vi "DRIVE_HDG_TARGET.vi"(10 "argv":string[](array[string]), 11 "args":u8) -> ()   [LabVIEW 2011]
uses:
  <vilib>/Rock Robotics/WPI/DriverStation/WPI_DriverStationStatusErrorCache.ctl
  Auto_Conf.vi
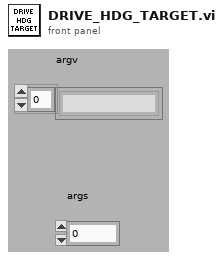
[diagram p1: front panel]
types:
  T1 = typedef "WPI_GyroDevRef.ctl" = cluster{"DevStatus":errorcluster, "Analog Module":T2, "Analog Channel":T3, "Offset":dbl, "Gain (VoltsPerDegree/Second)":dbl}
  T2 = typedef "FPGA_TypedefAnalogModule.ctl" = enum16{"Analog Module 1", "Analog Module 2"}
  T3 = typedef "FPGA_AIChannel.ctl" = enum8{"AI 1", "AI 2", "AI 3", "AI 4", "AI 5", "AI 6", "AI 7", "AI 8", "Invalid"}
  T4 = typedef "WPI_DriverStationStatusErrorCache.ctl" = enum16{"Get", "Set"}
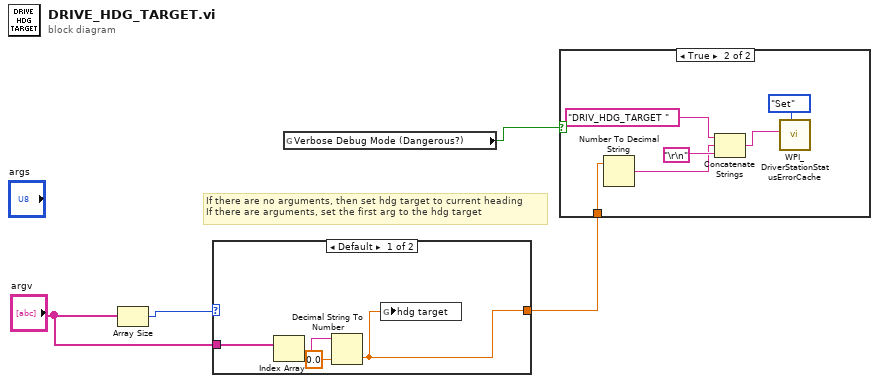
[diagram p0: block diagram]
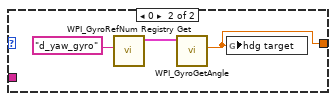
[diagram p3: hidden frame]
diagram:
  # "If there are no arguments, then set hdg target to current heading\nIf there are arguments, set the first arg to the hdg target"
  n1 = Array Size(array="argv") -> (size(s)=w1:i32)
  n2 = case shown="Default" w1 {
    tunnel: "argv" -> [w8 _]
    tunnel: [w5 w9] -> w3
    frame Default {
      n3 = Index Array(array=w8) -> (element=w7:string)  [unwired: 1 in]
      n4 = Decimal String To Number(string=w7, default (0L)=0.0 ("default (0 I32)")) -> (number=w5:dbl)  [unwired: 1 in, 1 out]
      n5 = global write "Auto_Conf.vi" "hdg target"(w5) -> ()
    }
    frame 0 {
      n6 = call <vilib>:"WPI_GyroRefNum Registry Get.vi"("refnum name"="d_yaw_gyro") -> ("GyroDevRef"=w10:T1)  [unwired: 1 in, 9 out]
      n7 = call <vilib>:"WPI_GyroGetAngle.vi"("GyroDevRef"=w10) -> ("Angle"=w9:dbl)  [unwired: 7 in, 3 out]
      n8 = global write "Auto_Conf.vi" "hdg target"(w9) -> ()
    }
  }
  n9 = global read "Auto_Conf.vi" "Verbose Debug Mode (Dangerous?)"() -> (w4:bool)
  n10 = case shown="True" w4 {
    tunnel: w3 -> [_ w12]
    frame False {
    }
    frame True {
      n11 = Number To Decimal String(number=w12) -> (decimal integer string=w13:string)  [unwired: 1 in]
      n12 = Concatenate Strings("DRIV_HDG_TARGET " ("string"), w13, "\r\n") -> (w15:string)
      n13 = call <vilib>:"WPI_DriverStationStatusErrorCache.vi"("StatusErrorCacheOp"=WPI_DriverStationStatusErrorCache."Set", "Error String"=w15) -> ()  [unwired: 10 out]
    }
  }
